vi "serialization tests.vi"() -> (0 "error out":errorcluster, 1 "lines access?":bool, 2 "modules access?":bool, 3 "channels access?":bool)   [LabVIEW 2014, in "Shared Memory tests.lvlib"]
doc: "Tests the 'To String' and 'From String' methods of the Module's configuration class and ensures they are compatible."
uses:
  Shared Memory tests.lvlib
  module/configuration/Shared Memory configuration.lvclass
  module/configuration/Shared Memory configuration.lvclass/Shared Memory configuration.ctl
  <vilib>/NI/Tag Bus Module Framework/channel/TBM channel.lvclass
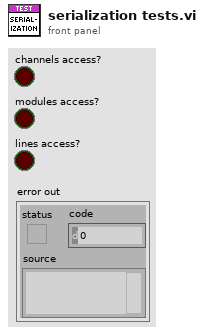
[diagram p1: front panel]
types:
  T1 = typedef "Shared Memory configuration.lvclass/Line.ctl" = cluster{"channel":refnum<class "TBM channel.lvclass">}
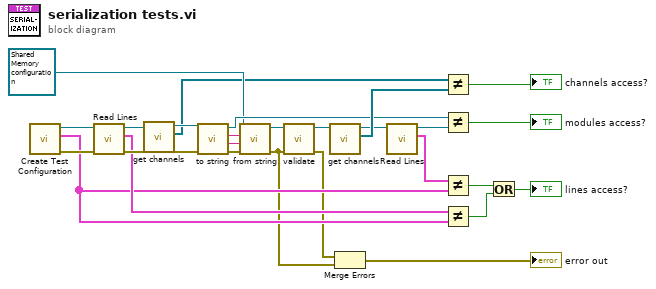
[diagram p0: block diagram]
diagram:
  n1 = call "Create Test Configuration.vi"() -> ("error out"=w12:errorcluster, "Lines"=w7:T1[], "Module Configuration"=w10:refnum<class "Shared Memory configuration.lvclass">)  [unwired: 3 in, 6 out]
  n2 = call "Read Lines.vi"("error in"=w12, "Shared Memory configuration in"=w10) -> ("error out"=w11:errorcluster, "Lines"=w8:T1[], "Shared Memory configuration out"=w9:refnum<class "Shared Memory configuration.lvclass">)  [unwired: 7 in]
  n3 = call-dynamic "get channels.vi"("Shared Memory configuration in"=w9) -> ("channels"=w16:refnum<class "TBM channel.lvclass">[], "Shared Memory configuration out"=w17:refnum<class "Shared Memory configuration.lvclass">)  [unwired: 9 in]
  n4 = call-dynamic "to string.vi"("error in"=w11, "Shared Memory configuration in"=w17) -> ("error out"=w27:errorcluster, "data"=w26:string, "version"=w25:string, "Shared Memory configuration out"=w19:refnum<class "Shared Memory configuration.lvclass">)  [unwired: 6 in]
  n5 = call-dynamic "from string.vi"("error in"=w27, "data"=w26, "version"=w25, "Shared Memory configuration in"=refnum<class "Shared Memory configuration.lvclass"> refnum ("tag bus configurable plugin module configuration")) -> ("error out"=w3:errorcluster, "Shared Memory configuration out"=w24:refnum<class "Shared Memory configuration.lvclass">)  [unwired: 6 in]
  n6 = call-dynamic "validate.vi"("error in"=w3, "Shared Memory configuration in"=w24) -> ("error out"=w2:errorcluster, "Shared Memory configuration out"=w22:refnum<class "Shared Memory configuration.lvclass">)  [unwired: 8 in]
  n7 = call-dynamic "get channels.vi"("Shared Memory configuration in"=w22) -> ("channels"=w21:refnum<class "TBM channel.lvclass">[], "Shared Memory configuration out"=w15:refnum<class "Shared Memory configuration.lvclass">)  [unwired: 9 in]
  n8 = Merge Errors(w2, w3) -> (→"error out":errorcluster)
  n9 = call "Read Lines.vi"("Shared Memory configuration in"=w15) -> ("Lines"=w13:T1[], "Shared Memory configuration out"=w14:refnum<class "Shared Memory configuration.lvclass">)  [unwired: 8 in, 1 out]
  n10 = Not Equal?(x=w16, y=w21) -> (x != y?=→"channels access?":bool)
  n11 = Not Equal?(x=w19, y=w14) -> (x != y?=→"modules access?":bool)
  n12 = Not Equal?(x=w13, y=w7) -> (x != y?=w5:bool)
  n13 = Not Equal?(x=w8, y=w7) -> (x != y?=w6:bool)
  n14 = Or(x=w5, y=w6) -> (x .or. y?=→"lines access?":bool)
